vi "Log.vi"(0 "object in":refnum<class "TDMS.lvclass">, 2 "Requirements":T2, 5 "Error In":errorcluster) -> (14 "object out":refnum<class "TDMS.lvclass">, 16 "Message":T1, 19 "Error Out":errorcluster)   [LabVIEW 2024, in "TDMS.lvclass"]
doc: "Open or grap already existing TDMS file and runs Logger classes Execute method"
uses:
  TDMS.lvclass
  Support/Type Def/Requirements.ctl
  Support/Type Def/File Type.ctl
  Support/Type Def/Message.ctl
  IDataMethod_interface/IDataMethod.lvclass
panel:
  # "Connector Pane"
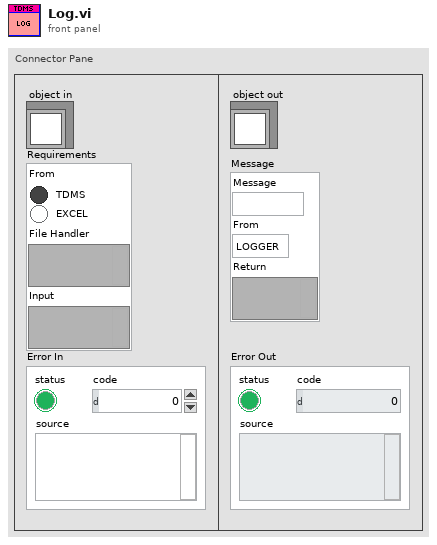
[diagram p1: front panel]
types:
  T1 = typedef "Message.ctl" = cluster{"Message":string, "From":enum16{"LOGGER", "VIEWER"}, "Return":variant}
  T2 = typedef "Requirements.ctl" = cluster{"From":T3, "File Handler":variant, "Input":variant}
  T3 = typedef "File Type.ctl" = enum32{"TDMS", "EXCEL"}
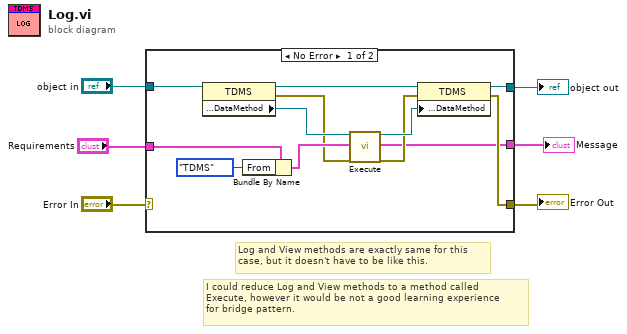
[diagram p0: block diagram]
diagram:
  # "I could reduce Log and View methods to a method called\nExecute, however it would be not a good learning experience\nfor bridge pattern."
  # "Log and View methods are exactly same for this\ncase, but it doesn't have to be like this."
  n1 = case shown="No Error" "Error In" {
    selector: "Error In" -> [_ w20]
    tunnel: [w8 w20] -> w5
    tunnel: [w13 w19] -> w3
    tunnel: "object in" -> [w15 w19]
    tunnel: "Requirements" -> [w11 _]
    tunnel: [w7 _] -> w1
    frame No Error {
      n2 = property class="TDMS"(reference=w15) -> (reference out=w14:refnum<class "TDMS.lvclass">, error out=w10:errorcluster, "properties:DataMethod"=w17:refnum<class "IDataMethod.lvclass">)  [unwired: 1 in]
      n3 = Bundle By Name(cluster=w11, "From"=enum16{"TDMS", "EXCEL"}."TDMS") -> (w12:T2)
      n4 = call-dynamic "Execute.vi"("object in"=w17, "Requirements"=w12, "Error In"=w10) -> ("object out"=w18:refnum<class "IDataMethod.lvclass">, "Message"=w7:T1, "Error Out"=w9:errorcluster)  [unwired: 14 in]
      n5 = property class="TDMS"(reference=w14, error in=w9, "properties:DataMethod"=w18) -> (reference out=w13:refnum<class "TDMS.lvclass">, error out=w8:errorcluster)
    }
    frame Error {
    }
  }
  "Error Out" <- w5
  "object out" <- w3
  "Message" <- w1
